vi "Calculate I2C Wave.vi"(8 "error in (no error)":errorcluster, 11 "Simulation in":refnum<class "Simulation.lvclass">) -> (0 "error out":errorcluster, 3 "Simulation out":refnum<class "Simulation.lvclass">)   [LabVIEW 2020, in "Generic I2C.lvlib" / "Simulation.lvclass"]
uses:
  Simulation.lvclass
  C:/Users/kaiser.asan/OneDrive - SolitonTechnologies/LabVIEW/29.SDLC - I2C Driver/I2C Module/I2C Controller Module/Class/Devices/Parent/Devices.lvclass
  Transmission Mode/Parent/TX Speed.lvclass
  Addressing Mode/Parent/Addressing Mode.lvclass
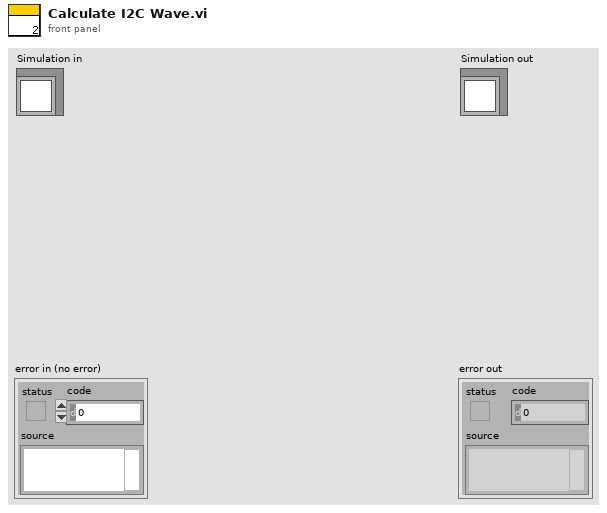
[diagram p1: front panel]
types:
  T1 = typedef "I2C Controller Lib.lvlib/Transmission Data.ctl" = u8[]
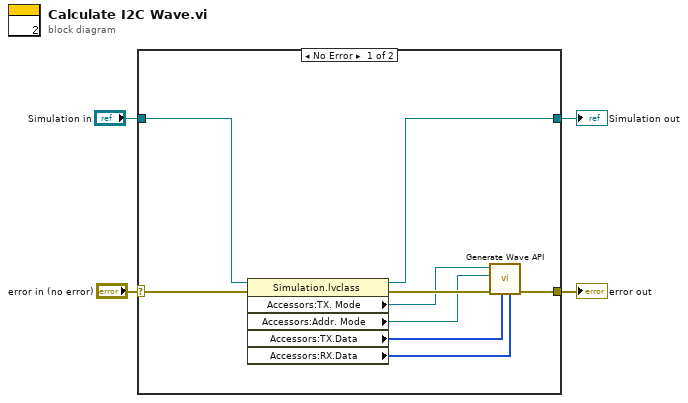
[diagram p0: block diagram]
diagram:
  n1 = case shown="No Error" "error in (no error)" {
    selector: "error in (no error)" -> [w13 w15]
    tunnel: [w8 w14] -> w1
    tunnel: "Simulation in" -> [w10 w14]
    tunnel: [w12 w15] -> w3
    frame No Error {
      n2 = property class="Simulation.lvclass"(reference=w10, error in=w13) -> (reference out=w8:refnum<class "Simulation.lvclass">, error out=w11:errorcluster, "Accessors:TX. Mode"=w9:refnum<data-value>, "Accessors:Addr. Mode"=w7:refnum<data-value>, "Accessors:TX.Data"=w6:T1, "Accessors:RX.Data"=w5:u8[])
      n3 = call "Generate Wave API.vi"("RX.Data"=w5, "TX.Data"=w6, "error in (no error)"=w11, "Addr. Mode"=w7, "DVR IN"=w9) -> ("error out"=w12:errorcluster)  [unwired: 5 in, 1 out]
    }
    frame Error {
      # "Error Found."
    }
  }
  "error out" <- w3
  "Simulation out" <- w1
